vi "About Dialog.vi"() -> ()   [LabVIEW 2020, in "Execution UI V2.lvclass"]
uses:
  Execution UI V2.lvclass
  Execution UI V2.lvclass/Execution UI V2.ctl
panel:
  in  "Refresh":bool
  in  "Run Single Test":bool
  in  "Stop":bool
  in  "Run All Tests":bool
  # "1"
  # "LUnit Unit Test Framework"
  # "MIT License\nCopyright © 2021 Astemes\nDeveloped by Anton Sundqvist\nEnabled by LabVIEW Community Edition\nPlease use VIPM to determine the currently installed version"
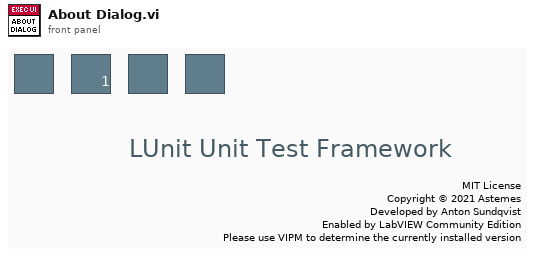
[diagram p1: front panel]
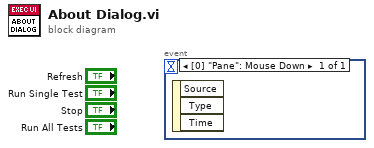
[diagram p0: block diagram]
diagram:
  n1 = event shown="[0] \"Pane\": Mouse Down" {
    selector: _ -> [_]
    dyn-events: _ -> [_]
    timeout: _ -> [_]
    event Mouse Down {
      n2 = event-data() -> ()  [unwired: 1 in, 3 out]
    }
  }
